vi "Swerve_test.vi"(9 "indeadzone":bool, 10 "Encoder":dbl, 11 "Joystick":dbl) -> (2 "Return":dbl)   [LabVIEW 2016]
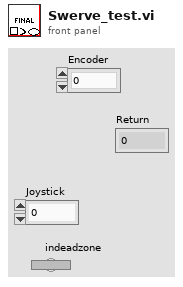
[diagram p1: front panel]
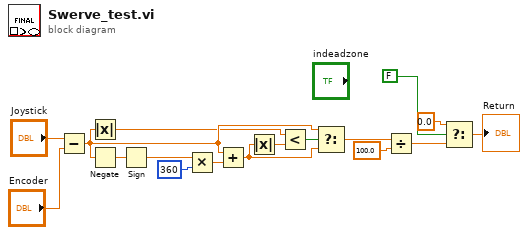
[diagram p0: block diagram]
diagram:
  n1 = Subtract(x="Joystick", y="Encoder") -> (x-y=w8:dbl)
  n2 = Absolute Value(x=w8) -> (abs(x)=w7:dbl)
  n3 = Negate(x=w8) -> (-x=w13:dbl)
  n4 = Sign(1:w13) -> (0:w12:dbl)
  n5 = Multiply(x=w12, y=360) -> (x*y=w11:dbl)
  n6 = Add(x=w8, y=w11) -> (x+y=w10:dbl)
  n7 = Absolute Value(x=w10) -> (abs(x)=w9:dbl)
  n8 = Less?(x=w7, y=w9) -> (x < y?=w15:bool)
  n9 = Select(t=w8, s=w15, f=w10) -> (s? t:f=w3:dbl)
  n10 = Divide(x=w3, y=100.0) -> (x/y=w4:dbl)
  n11 = Select(t=0.0, s=FALSE, f=w4) -> (s? t:f=→"Return":dbl)
